vi "Read Multiple Parameters.vi"(7 "Single Lock-in Parameter 3 (-1: None)":i32(ring)=-1 items=["None"=-1, "X output"=0, "Y output"=1, "R output"=2, "Theta output"=3, "Aux In 1"=4, "Aux In 2"=5, "Aux In 3"=6, "Aux In 4"=7, "Aux Out 1"=8, "Aux Out 2"=9, "Xnoise"=10, "Ynoise"=11, "Reference Phase"=12, "Sine Out Amplitude"=13, "DC Level"=14, "Int. Ref. Frequency"=15, "Ext. Ref. Frequency"=16], 8 "error in (no error)":errorcluster, 9 "Single Lock-in Parameter 2 (0: X output)":i32(ring) items=["X output", "Y output", "R output", "Theta output", "Aux In 1", "Aux In 2", "Aux In 3", "Aux In 4", "Aux Out 1", "Aux Out 2", "Xnoise", "Ynoise", "Reference Phase", "Sine Out Amplitude", "DC Level", "Int. Ref. Frequency", "Ext. Ref. Frequency"], 10 "Single Lock-in Parameter 1 (0: X output)":i32(ring) items=["X output", "Y output", "R output", "Theta output", "Aux In 1", "Aux In 2", "Aux In 3", "Aux In 4", "Aux Out 1", "Aux Out 2", "Xnoise", "Ynoise", "Reference Phase", "Sine Out Amplitude", "DC Level", "Int. Ref. Frequency", "Ext. Ref. Frequency"], 11 "VISA resource name":refnum<visa-resource-name>) -> (1 "Output Value(3 parameters)":T1, 2 "Output Value(2 parameters)":cluster{"Value 1":dbl, "Value 2":dbl}, 3 "VISA resource name out":refnum<visa-resource-name>)   [LabVIEW 2020, in "Stanford Research SR865.lvlib"]
doc: "Reads all the available parameters from the instrument.\n\n<b>Note:</b>\nThis VI only reads multiple parameters, not multiple points of the same parameter."
uses:
  Stanford Research SR865.lvlib
panel:
  # "Required Generator"
  # "Optional Generator"
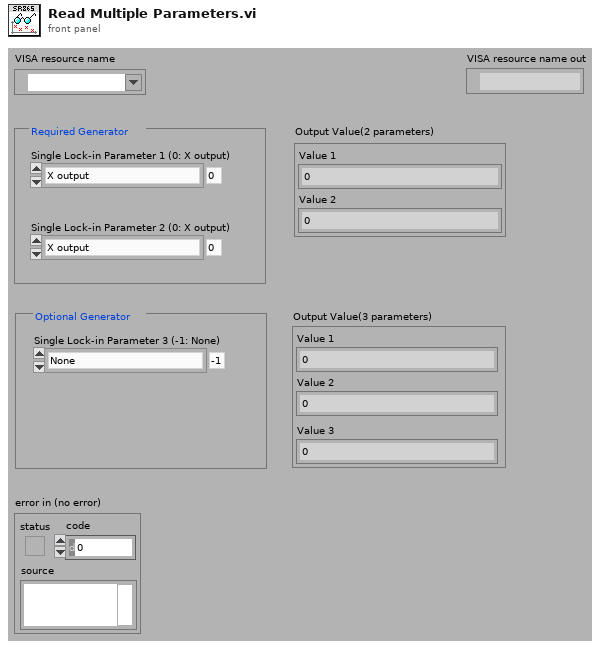
[diagram p1: front panel]
types:
  T1 = cluster{"Value 1":dbl, "Value 2":dbl, "Value 3":dbl}
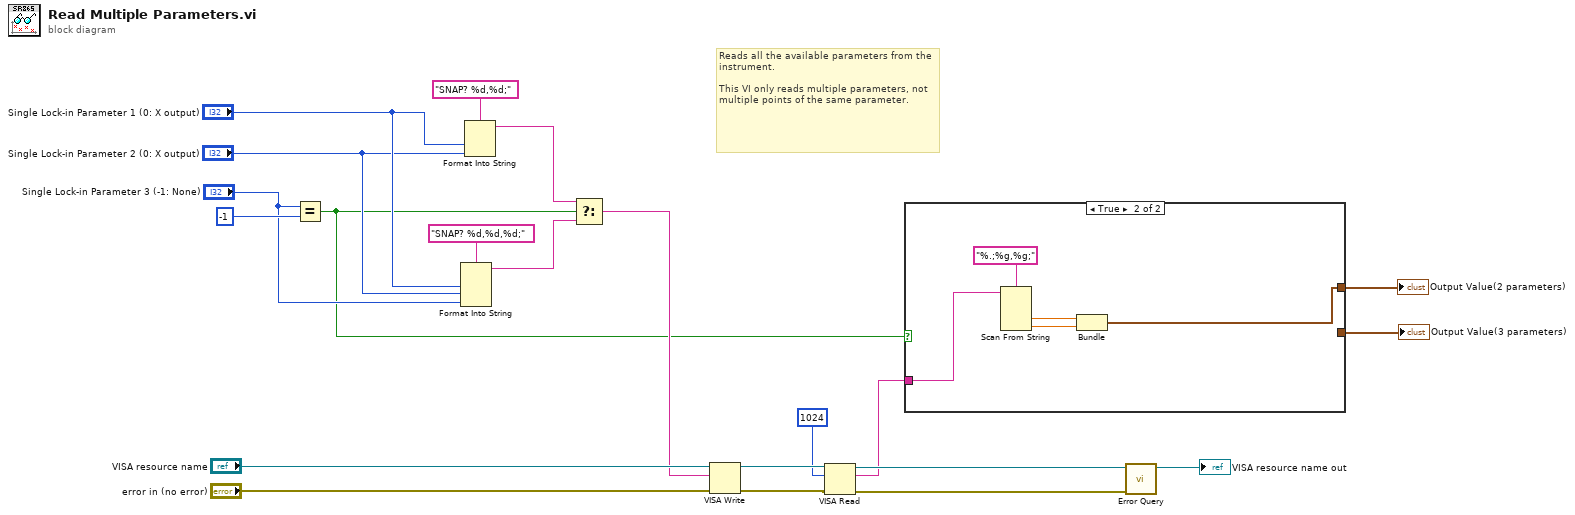
[diagram p0: block diagram]
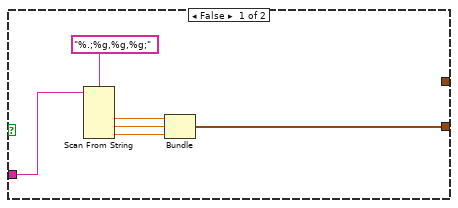
[diagram p2: hidden frame]
diagram:
  # "Reads all the available parameters from the instrument.\n\nThis VI only reads multiple parameters, not multiple points of the same parameter."
  n1 = Equal?(x="Single Lock-in Parameter 3 (-1: None)", y=-1) -> (x = y?=w4:bool)
  n2 = Format Into String(format string="SNAP? %d,%d,%d;", "Single Lock-in Parameter 1 (0: X output)", "Single Lock-in Parameter 2 (0: X output)", "Single Lock-in Parameter 3 (-1: None)") -> (resulting string=w10:string)  [unwired: 2 in, 1 out]
  n3 = Format Into String(format string="SNAP? %d,%d;", "Single Lock-in Parameter 1 (0: X output)", "Single Lock-in Parameter 2 (0: X output)") -> (resulting string=w9:string)  [unwired: 2 in, 1 out]
  n4 = Select(t=w9, s=w4, f=w10) -> (s? t:f=w8:string)
  n5 = VISA Write(VISA resource name="VISA resource name", write buffer=w8, error in (no error)="error in (no error)") -> (VISA resource name out=w17:refnum<visa-resource-name>, error out=w15:errorcluster)  [unwired: 1 out]
  n6 = VISA Read(VISA resource name=w17, byte count=u32 1024, error in (no error)=w15) -> (VISA resource name out=w16:refnum<visa-resource-name>, read buffer=w3:string, error out=w14:errorcluster)  [unwired: 1 out]
  n7 = case shown="True" w4 {
    tunnel: w3 -> [w23 w29]
    tunnel: [w22 _] -> w2
    tunnel: [_ w28] -> w1
    frame False {
      n8 = Scan From String(format string="%.;%g,%g,%g;", input string=w23) -> (output 1=w25:dbl, output 2=w26:dbl, output 3=w27:dbl)  [unwired: 5 in, 3 out]
      n9 = Bundle(w25, w26, w27) -> (w22:cluster{dbl, dbl, dbl})  [unwired: 1 in]
    }
    frame True {
      n10 = Scan From String(format string="%.;%g,%g;", input string=w29) -> (output 1=w31:dbl, output 2=w32:dbl)  [unwired: 4 in, 3 out]
      n11 = Bundle(w31, w32) -> (w28:cluster{dbl, dbl})  [unwired: 1 in]
    }
  }
  "Output Value(3 parameters)" <- w2
  "Output Value(2 parameters)" <- w1
  n12 = call "Error Query.vi"("error in (no error)"=w14, "VISA resource name"=w16) -> ("VISA resource name out"=→"VISA resource name out":refnum<visa-resource-name>)  [unwired: 7 in, 2 out]
